vi "Read Last Measurement.vi"(8 "error in (no error)":errorcluster, 11 "VISA resource name":refnum<visa-resource-name>) -> (0 "error out":errorcluster, 2 "Last Data":dbl, 3 "VISA resource name out":refnum<visa-resource-name>)   [LabVIEW 2013, in "Agilent 3446X Series.lvlib"]
doc: "Returns the last measurement taken."
uses:
  <instrlib>/Agilent 3446X Series/Agilent 3446X Series.lvlib
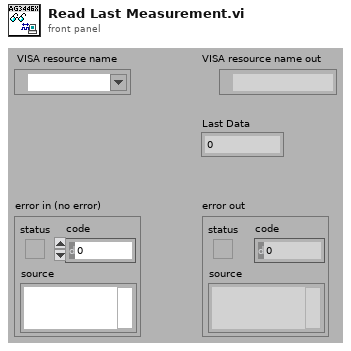
[diagram p1: front panel]
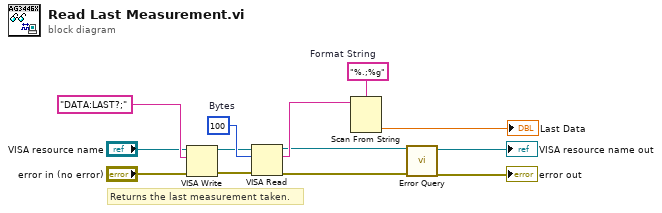
[diagram p0: block diagram]
diagram:
  w7 = "%.;%g"  # Format String
  w8 = u32 100  # Bytes
  # "Returns the last measurement taken."
  n1 = VISA Write(VISA resource name="VISA resource name", write buffer="DATA:LAST?;", error in (no error)="error in (no error)") -> (VISA resource name out=w4:refnum<visa-resource-name>, error out=w1:errorcluster)  [unwired: 1 out]
  n2 = VISA Read(VISA resource name=w4, byte count=w8, error in (no error)=w1) -> (VISA resource name out=w3:refnum<visa-resource-name>, read buffer=w6:string, error out=w2:errorcluster)  [unwired: 1 out]
  n3 = Scan From String(format string=w7, input string=w6) -> (output 1=→"Last Data":dbl)  [unwired: 2 in, 4 out]
  n4 = call <instrlib>:"Error Query.vi"("error in (no error)"=w2, "VISA resource name"=w3) -> ("error out"=→"error out":errorcluster, "VISA resource name out"=→"VISA resource name out":refnum<visa-resource-name>)  [unwired: 8 out]
